vi "NI5112.ProcCases.vi"(0 "i ref in":refnum<vi>, 1 "selector":string, 2 "Data":T1, 3 "call cluster":T2={"Object"="", "Selector"="", "CallType"=enum."synchronous", "Async Object"="", "Async Selector"="", "Data Descriptor"="", "Data"=[], "Error #"=0, "Expire"=0}, 5 "error in (no error)":errorcluster) -> (14 "i ref out":refnum<vi>, 17 "answer cluster":T2={"Object"="", "Selector"="", "CallType"=enum."synchronous", "Async Object"="", "Async Selector"="", "Data Descriptor"="", "Data"=[], "Error #"=0, "Expire"=0}, 19 "error out":errorcluster)   [LabVIEW 2014, in "NI5112.lvlib"]
doc: "This method is called by a process from within the default case in the event loop. The methods of a class that are linked to events will be called from THIS method. Add your code here."
uses:
  NI5112.lvlib
  CS_Core/CSSystem/CoreDefs/CoreDefs.call_type.ctl
  CS_Core/BaseProcess/BaseProcess.descriptor string definition.ctl
  CS_Core/CSSystem/CoreDefs/CoreDefs.rawDataType.ctl
  CS_Core/CSSystem/CoreLib/CoreLib.string 2 byte array.vi
  CS_Core/CSSystem/CoreLib/CoreLib.int 2 byte array.vi
  CS_Core/CSSystem/CoreLib/CoreLib.byte array 2 string.vi
  CS_Core/CSSystem/CoreLib/CoreLib.byte array 2 double.vi
  CS_Core/CSSystem/CoreLib/CoreLib.byte array 2 int.vi
  CS_Core/CSSystem/CoreLib/CoreLib.double 2 byte array.vi
  CS_Core/CSSystem/CoreLib/CoreLib.double array 2 byte array.vi
  CS_Core/BaseProcess/BaseProcess.lvlib
  CS_Core/CSSystem/CoreLib/CoreLib.lvlib
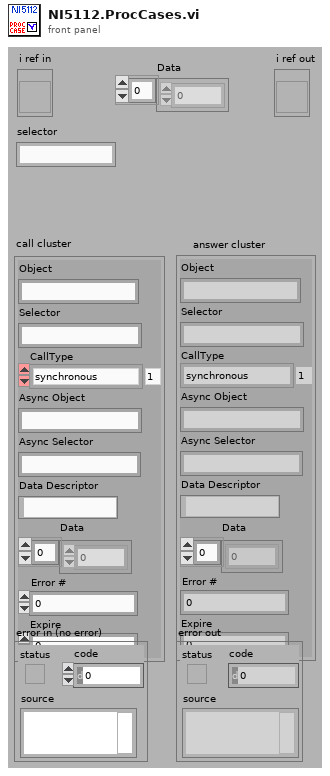
[diagram p1: front panel]
types:
  T1 = typedef "CoreDefs.rawDataType.ctl" = i8[]
  T2 = typedef "CoreDefs.call_type.ctl" = cluster{"Object":string, "Selector":string, "CallType":enum16{"simple", "synchronous", "asynchronous"}, "Async Object":string, "Async Selector":string, "Data Descriptor":T3, "Data":T1, "Error #":i32, "Expire":u32}
  T3 = typedef "BaseProcess.lvlib/BaseProcess.descriptor string definition.ctl" = string
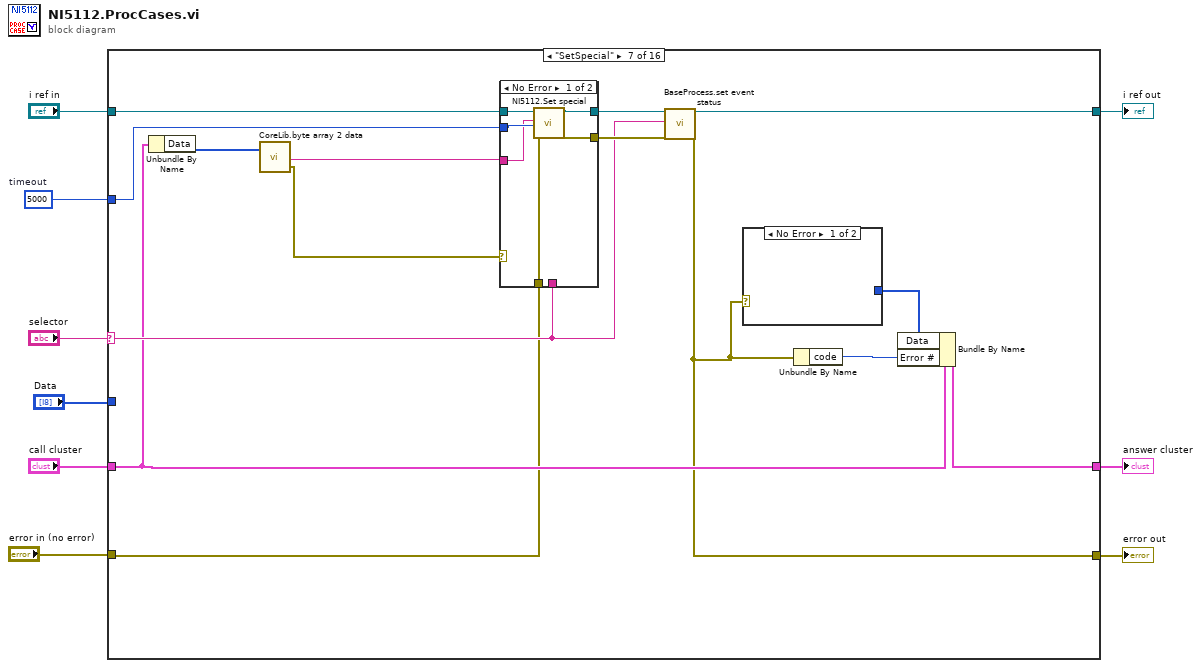
[diagram p0: block diagram]
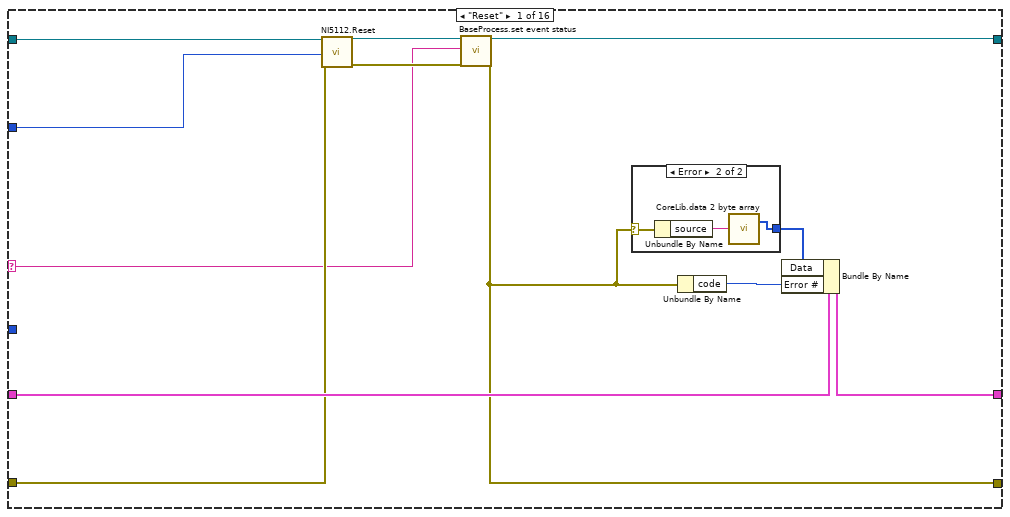
[diagram p2: hidden frame]
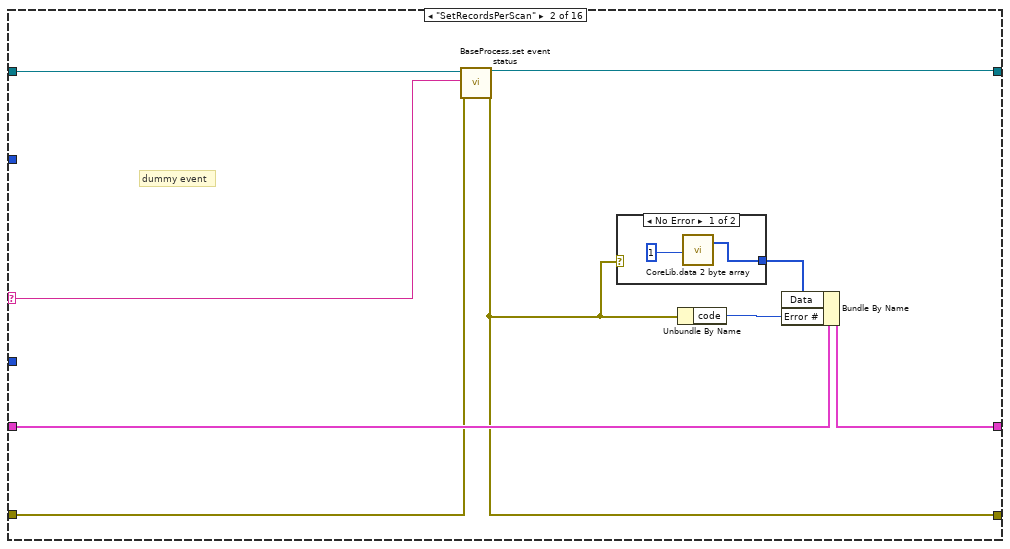
[diagram p4: hidden frame]
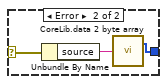
[diagram p5: hidden frame]
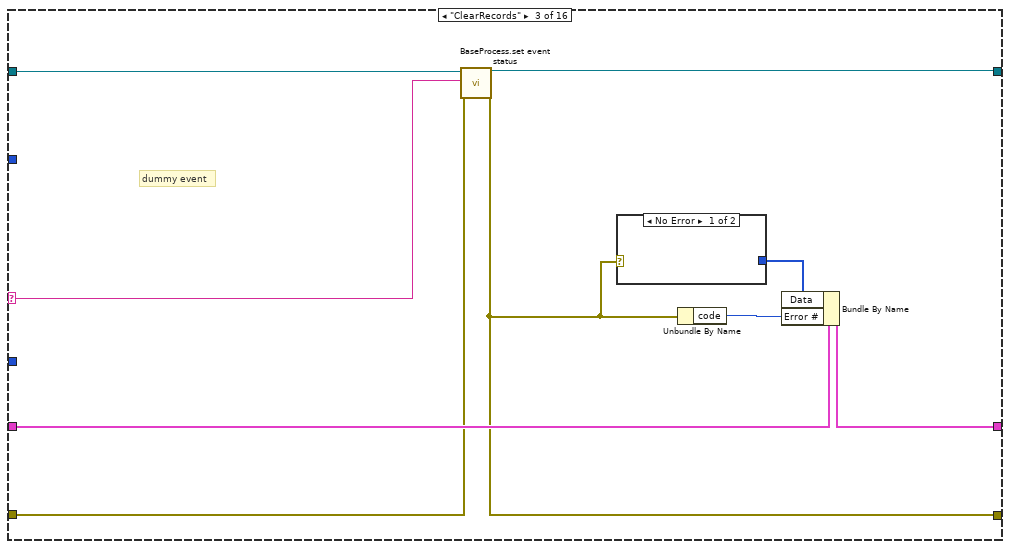
[diagram p6: hidden frame]
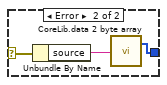
[diagram p7: hidden frame]
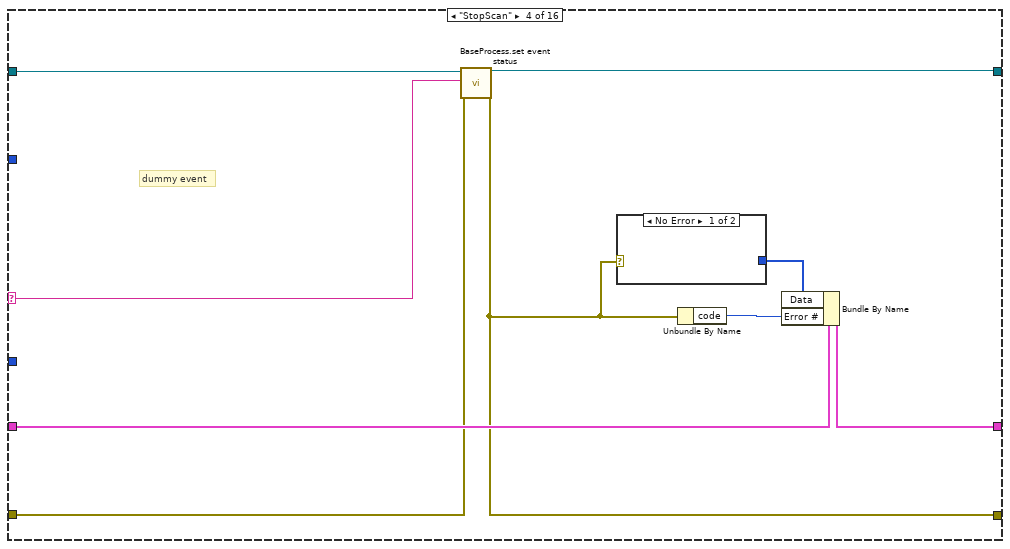
[diagram p8: hidden frame]
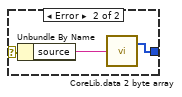
[diagram p9: hidden frame]
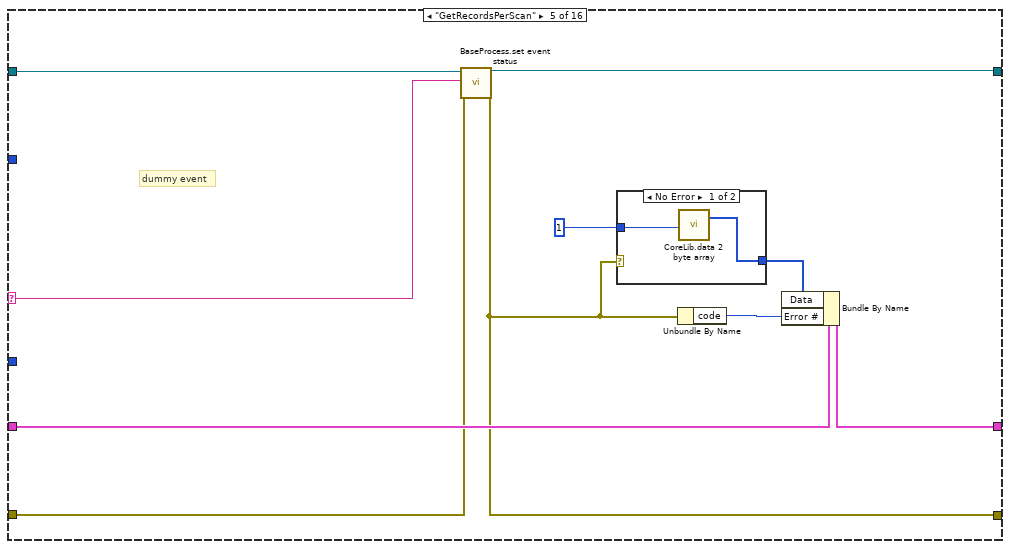
[diagram p10: hidden frame]
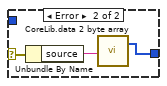
[diagram p11: hidden frame]
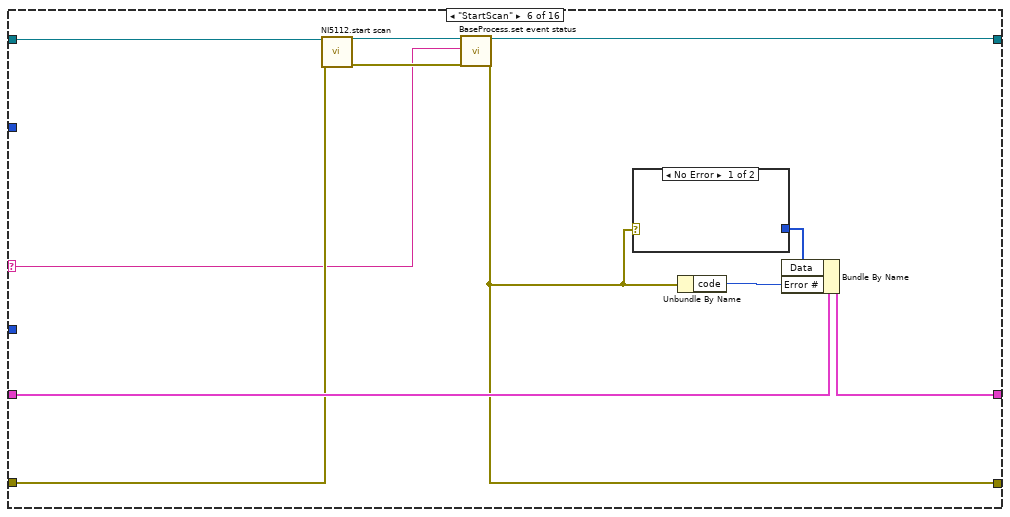
[diagram p12: hidden frame]
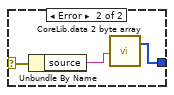
[diagram p13: hidden frame]
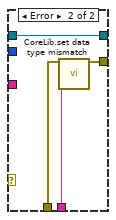
[diagram p14: hidden frame]
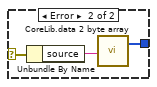
[diagram p15: hidden frame]
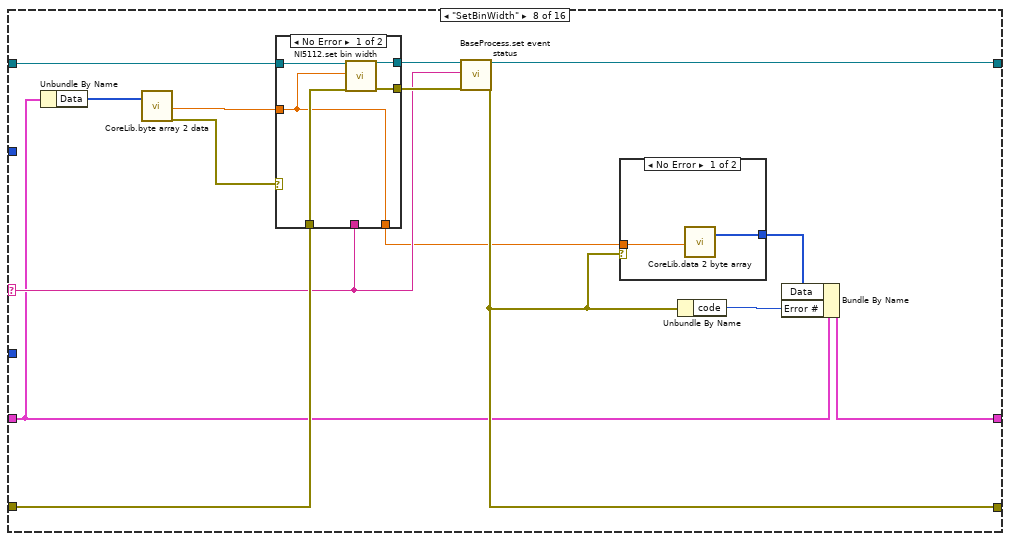
[diagram p16: hidden frame]
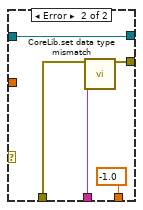
[diagram p17: hidden frame]
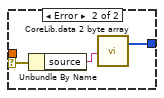
[diagram p18: hidden frame]
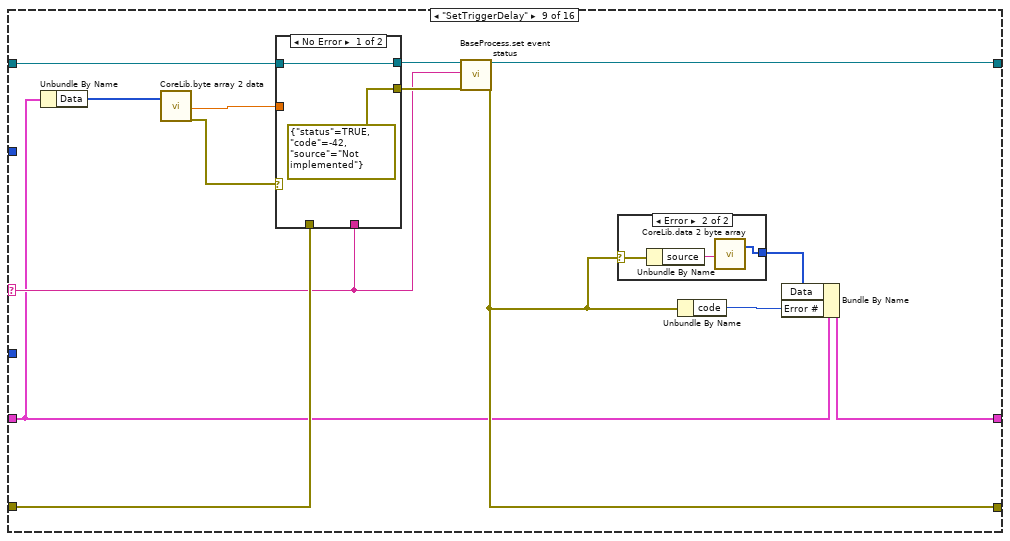
[diagram p19: hidden frame]
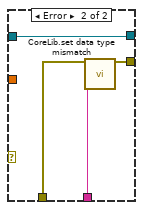
[diagram p20: hidden frame]
diagram:
  w2 = 5000  # timeout
  n1 = case shown="\"SetSpecial\"" "selector" {
    selector: "selector" -> [w11 w26 w40 w52 w65 w78 w100 w125 w154 w178 w205 w223 w243 w265 w282 w298]
    tunnel: "Data" -> [_ _ _ _ _ _ _ _ _ _ _ _ _ _ _ w297]
    tunnel: "i ref in" -> [w17 w25 w39 w51 w64 w84 w102 w131 w160 w184 w211 w229 w249 w271 w288 w304]
    tunnel: [w14 w29 w43 w55 w68 w81 w101 w128 w157 w181 w208 w226 w246 w268 w285 w303] -> w8
    tunnel: "call cluster" -> [w21 w33 w47 w59 w72 w88 w99 w124 w153 w177 w204 w222 w242 w264 w281 w299]
    tunnel: [w20 w32 w46 w58 w71 w87 w96 w134 w163 w187 w214 w232 w251 w274 w291 w300] -> w4
    tunnel: "error in (no error)" -> [w16 w28 w42 w54 w67 w83 w98 w130 w159 w183 w210 w228 w248 w270 w287 w302]
    tunnel: [w12 w27 w41 w53 w66 w79 w97 w126 w155 w179 w206 w224 w244 w266 w283 w301] -> w3
    tunnel: w2 -> [w10 _ _ _ _ _ w95 _ _ _ _ _ _ _ _ _]
    frame "Reset" {
      n2 = call "NI5112.Reset.vi"("i ref in"=w17, "ms timeout (100)"=w10, "error in (no error)"=w16) -> ("i ref out"=w15:refnum<vi>, "error out"=w13:errorcluster)  [unwired: 14 in, 1 out]
      n3 = call "BaseProcess.set event status.vi"("i ref in"=w15, "EventStatus"=w11, "error in (no error)"=w13) -> ("i ref out"=w14:refnum<vi>, "error out"=w12:errorcluster)  [unwired: 14 in, 1 out]
      n4 = case shown="Error" w12 {
        selector: w12 -> [_ w24]
        tunnel: [_ w22] -> w18
        frame No Error {
        }
        frame Error {
          n5 = Unbundle By Name(w24) -> ("source"=w23:string)
          n6 = call-poly "CoreLib.data 2 byte array.vi"("string"=w23) -> ("byteArray out"=w22:T1)  [unwired: 18 in]
        }
      }
      n7 = Unbundle By Name(w12) -> ("code"=w19:i32)
      n8 = Bundle By Name(cluster=w21, "Data"=w18, "Error #"=w19) -> (w20:T2)
    }
    frame "SetRecordsPerScan" {
      # "dummy event"
      n9 = call "BaseProcess.set event status.vi"("i ref in"=w25, "EventStatus"=w26, "error in (no error)"=w28) -> ("i ref out"=w29:refnum<vi>, "error out"=w27:errorcluster)  [unwired: 14 in, 1 out]
      n10 = case shown="No Error" w27 {
        selector: w27 -> [_ w38]
        tunnel: [w34 w36] -> w30
        frame No Error {
          n11 = call-poly "CoreLib.data 2 byte array.vi"("i32"=1) -> ("byteArray out"=w34:T1)  [unwired: 18 in]
        }
        frame Error {
          n12 = Unbundle By Name(w38) -> ("source"=w37:string)
          n13 = call-poly "CoreLib.data 2 byte array.vi"("string"=w37) -> ("byteArray out"=w36:T1)  [unwired: 18 in]
        }
      }
      n14 = Unbundle By Name(w27) -> ("code"=w31:i32)
      n15 = Bundle By Name(cluster=w33, "Data"=w30, "Error #"=w31) -> (w32:T2)
    }
    frame "ClearRecords" {
      # "dummy event"
      n16 = call "BaseProcess.set event status.vi"("i ref in"=w39, "EventStatus"=w40, "error in (no error)"=w42) -> ("i ref out"=w43:refnum<vi>, "error out"=w41:errorcluster)  [unwired: 14 in, 1 out]
      n17 = case shown="No Error" w41 {
        selector: w41 -> [_ w50]
        tunnel: [_ w48] -> w44
        frame No Error {
        }
        frame Error {
          n18 = Unbundle By Name(w50) -> ("source"=w49:string)
          n19 = call-poly "CoreLib.data 2 byte array.vi"("string"=w49) -> ("byteArray out"=w48:T1)  [unwired: 18 in]
        }
      }
      n20 = Unbundle By Name(w41) -> ("code"=w45:i32)
      n21 = Bundle By Name(cluster=w47, "Data"=w44, "Error #"=w45) -> (w46:T2)
    }
    frame "StopScan" {
      # "dummy event"
      n22 = call "BaseProcess.set event status.vi"("i ref in"=w51, "EventStatus"=w52, "error in (no error)"=w54) -> ("i ref out"=w55:refnum<vi>, "error out"=w53:errorcluster)  [unwired: 14 in, 1 out]
      n23 = case shown="No Error" w53 {
        selector: w53 -> [_ w62]
        tunnel: [_ w60] -> w56
        frame No Error {
        }
        frame Error {
          n24 = Unbundle By Name(w62) -> ("source"=w61:string)
          n25 = call-poly "CoreLib.data 2 byte array.vi"("string"=w61) -> ("byteArray out"=w60:T1)  [unwired: 18 in]
        }
      }
      n26 = Unbundle By Name(w53) -> ("code"=w57:i32)
      n27 = Bundle By Name(cluster=w59, "Data"=w56, "Error #"=w57) -> (w58:T2)
    }
    frame "GetRecordsPerScan" {
      # "dummy event"
      n28 = call "BaseProcess.set event status.vi"("i ref in"=w64, "EventStatus"=w65, "error in (no error)"=w67) -> ("i ref out"=w68:refnum<vi>, "error out"=w66:errorcluster)  [unwired: 14 in, 1 out]
      n29 = case shown="No Error" w66 {
        selector: w66 -> [_ w77]
        tunnel: [w73 w75] -> w69
        tunnel: 1 -> [w74 _]
        frame No Error {
          n30 = call-poly "CoreLib.data 2 byte array.vi"("i32"=w74) -> ("byteArray out"=w73:T1)  [unwired: 18 in]
        }
        frame Error {
          n31 = Unbundle By Name(w77) -> ("source"=w76:string)
          n32 = call-poly "CoreLib.data 2 byte array.vi"("string"=w76) -> ("byteArray out"=w75:T1)  [unwired: 18 in]
        }
      }
      n33 = Unbundle By Name(w66) -> ("code"=w70:i32)
      n34 = Bundle By Name(cluster=w72, "Data"=w69, "Error #"=w70) -> (w71:T2)
    }
    frame "StartScan" {
      n35 = call "NI5112.start scan.vi"("i ref in"=w84, "error in (no error)"=w83) -> ("i ref out"=w82:refnum<vi>, "error out"=w80:errorcluster)  [unwired: 15 in, 1 out]
      n36 = call "BaseProcess.set event status.vi"("i ref in"=w82, "EventStatus"=w78, "error in (no error)"=w80) -> ("i ref out"=w81:refnum<vi>, "error out"=w79:errorcluster)  [unwired: 14 in, 1 out]
      n37 = case shown="No Error" w79 {
        selector: w79 -> [_ w91]
        tunnel: [_ w89] -> w85
        frame No Error {
        }
        frame Error {
          n38 = Unbundle By Name(w91) -> ("source"=w90:string)
          n39 = call-poly "CoreLib.data 2 byte array.vi"("string"=w90) -> ("byteArray out"=w89:T1)  [unwired: 18 in]
        }
      }
      n40 = Unbundle By Name(w79) -> ("code"=w86:i32)
      n41 = Bundle By Name(cluster=w88, "Data"=w85, "Error #"=w86) -> (w87:T2)
    }
    frame "SetSpecial" {
      n42 = Unbundle By Name(w99) -> ("Data"=w94:T1)
      n43 = call-poly "CoreLib.byte array 2 data.vi"("byteArray"=w94) -> ("string"=w93:string, "error out"=w92:errorcluster)  [unwired: 16 in, 1 out]
      n44 = case shown="No Error" w92 {
        tunnel: w98 -> [w110 w115]
        tunnel: [w111 w113] -> w104
        tunnel: [w112 w116] -> w103
        tunnel: w100 -> [_ w114]
        tunnel: w93 -> [w107 _]
        tunnel: w95 -> [w109 _]
        tunnel: w102 -> [w108 w113]
        frame No Error {
          n45 = call "NI5112.Set special.vi"("i ref in"=w108, "Special"=w107, "ms timeout (100)"=w109, "error in (no error)"=w110) -> ("i ref out"=w111:refnum<vi>, "error out"=w112:errorcluster)  [unwired: 13 in, 1 out]
        }
        frame Error {
          n46 = call "CoreLib.set data type mismatch.vi"("error in (no error)"=w115, "error source"=w114) -> ("error out"=w116:errorcluster)  [unwired: 17 in]
        }
      }
      n47 = call "BaseProcess.set event status.vi"("i ref in"=w104, "EventStatus"=w100, "error in (no error)"=w103) -> ("i ref out"=w101:refnum<vi>, "error out"=w97:errorcluster)  [unwired: 14 in, 1 out]
      n48 = case shown="No Error" w97 {
        selector: w97 -> [_ w119]
        tunnel: [_ w117] -> w105
        frame No Error {
        }
        frame Error {
          n49 = Unbundle By Name(w119) -> ("source"=w118:string)
          n50 = call-poly "CoreLib.data 2 byte array.vi"("string"=w118) -> ("byteArray out"=w117:T1)  [unwired: 18 in]
        }
      }
      n51 = Unbundle By Name(w97) -> ("code"=w106:i32)
      n52 = Bundle By Name(cluster=w99, "Data"=w105, "Error #"=w106) -> (w96:T2)
    }
    frame "SetBinWidth" {
      n53 = Unbundle By Name(w124) -> ("Data"=w120:T1)
      n54 = call-poly "CoreLib.byte array 2 data.vi"("byteArray"=w120) -> ("d64"=w122:dbl, "error out"=w121:errorcluster)  [unwired: 16 in, 1 out]
      n55 = case shown="No Error" w121 {
        tunnel: w131 -> [w139 w141]
        tunnel: w130 -> [w138 w143]
        tunnel: [w137 w141] -> w129
        tunnel: [w136 w144] -> w127
        tunnel: w125 -> [_ w142]
        tunnel: w122 -> [w135 _]
        tunnel: [w135 -1.0 ("act bin width")] -> w123
        frame No Error {
          n56 = call "NI5112.set bin width.vi"("i ref in"=w139, "bin width [us]"=w135, "error in (no error)"=w138) -> ("i ref out"=w137:refnum<vi>, "error out"=w136:errorcluster)  [unwired: 14 in, 1 out]
        }
        frame Error {
          n57 = call "CoreLib.set data type mismatch.vi"("error in (no error)"=w143, "error source"=w142) -> ("error out"=w144:errorcluster)  [unwired: 17 in]
        }
      }
      n58 = call "BaseProcess.set event status.vi"("i ref in"=w129, "EventStatus"=w125, "error in (no error)"=w127) -> ("i ref out"=w128:refnum<vi>, "error out"=w126:errorcluster)  [unwired: 14 in, 1 out]
      n59 = case shown="No Error" w126 {
        selector: w126 -> [_ w149]
        tunnel: [w145 w148] -> w132
        tunnel: w123 -> [w146 _]
        frame No Error {
          n60 = call-poly "CoreLib.data 2 byte array.vi"("i32"=w146) -> ("byteArray out"=w145:T1)  [unwired: 18 in]
        }
        frame Error {
          n61 = Unbundle By Name(w149) -> ("source"=w147:string)
          n62 = call-poly "CoreLib.data 2 byte array.vi"("string"=w147) -> ("byteArray out"=w148:T1)  [unwired: 18 in]
        }
      }
      n63 = Unbundle By Name(w126) -> ("code"=w133:i32)
      n64 = Bundle By Name(cluster=w124, "Data"=w132, "Error #"=w133) -> (w134:T2)
    }
    frame "SetTriggerDelay" {
      n65 = Unbundle By Name(w153) -> ("Data"=w151:T1)
      n66 = call-poly "CoreLib.byte array 2 data.vi"("byteArray"=w151) -> ("d64"=w152:dbl, "error out"=w150:errorcluster)  [unwired: 16 in, 1 out]
      n67 = case shown="No Error" w150 {
        tunnel: w160 -> [w164 w166]
        tunnel: w159 -> [_ w168]
        tunnel: [w164 w166] -> w158
        tunnel: [errorcluster {"status"=TRUE, "code"=-42, "source"="Not implemented"} ("error out") w169] -> w156
        tunnel: w154 -> [_ w167]
        tunnel: w152 -> [_ _]
        frame No Error {
        }
        frame Error {
          n68 = call "CoreLib.set data type mismatch.vi"("error in (no error)"=w168, "error source"=w167) -> ("error out"=w169:errorcluster)  [unwired: 17 in]
        }
      }
      n69 = call "BaseProcess.set event status.vi"("i ref in"=w158, "EventStatus"=w154, "error in (no error)"=w156) -> ("i ref out"=w157:refnum<vi>, "error out"=w155:errorcluster)  [unwired: 14 in, 1 out]
      n70 = case shown="Error" w155 {
        selector: w155 -> [_ w172]
        tunnel: [_ w170] -> w161
        frame No Error {
        }
        frame Error {
          n71 = Unbundle By Name(w172) -> ("source"=w171:string)
          n72 = call-poly "CoreLib.data 2 byte array.vi"("string"=w171) -> ("byteArray out"=w170:T1)  [unwired: 18 in]
        }
      }
      n73 = Unbundle By Name(w155) -> ("code"=w162:i32)
      n74 = Bundle By Name(cluster=w153, "Data"=w161, "Error #"=w162) -> (w163:T2)
    }
    frame "SetBinsPerRecord" {
      n75 = Unbundle By Name(w177) -> ("Data"=w175:T1)
      n76 = call-poly "CoreLib.byte array 2 data.vi"("byteArray"=w175) -> ("i32"=w174:i32, "error out"=w173:errorcluster)  [unwired: 16 in, 1 out]
      n77 = case shown="No Error" w173 {
        tunnel: w184 -> [w192 w194]
        tunnel: w183 -> [w191 w196]
        tunnel: [w190 w194] -> w182
        tunnel: [w189 w197] -> w180
        tunnel: w178 -> [_ w195]
        tunnel: w174 -> [w188 _]
        tunnel: [w188 -1 ("act bins per recored")] -> w176
        frame No Error {
          n78 = call "NI5112.SetBinsPerRecord.vi"("i ref in"=w192, "bins per record"=w188, "error in (no error)"=w191) -> ("i ref out"=w190:refnum<vi>, "error out"=w189:errorcluster)  [unwired: 14 in, 1 out]
        }
        frame Error {
          n79 = call "CoreLib.set data type mismatch.vi"("error in (no error)"=w196, "error source"=w195) -> ("error out"=w197:errorcluster)  [unwired: 17 in]
        }
      }
      n80 = call "BaseProcess.set event status.vi"("i ref in"=w182, "EventStatus"=w178, "error in (no error)"=w180) -> ("i ref out"=w181:refnum<vi>, "error out"=w179:errorcluster)  [unwired: 14 in, 1 out]
      n81 = case shown="No Error" w179 {
        selector: w179 -> [_ w202]
        tunnel: [w198 w200] -> w185
        tunnel: w176 -> [w199 _]
        frame No Error {
          n82 = call-poly "CoreLib.data 2 byte array.vi"("i32"=w199) -> ("byteArray out"=w198:T1)  [unwired: 18 in]
        }
        frame Error {
          n83 = Unbundle By Name(w202) -> ("source"=w201:string)
          n84 = call-poly "CoreLib.data 2 byte array.vi"("string"=w201) -> ("byteArray out"=w200:T1)  [unwired: 18 in]
        }
      }
      n85 = Unbundle By Name(w179) -> ("code"=w186:i32)
      n86 = Bundle By Name(cluster=w177, "Data"=w185, "Error #"=w186) -> (w187:T2)
    }
    frame "GetScanStatus" {
      n87 = call "NI5112.get scan status.vi"("i ref in"=w211, "error in (no error)"=w210) -> ("i ref out"=w209:refnum<vi>, "x != y?"=w203:bool, "error out"=w207:errorcluster)  [unwired: 14 in, 1 out]
      n88 = call "BaseProcess.set event status.vi"("i ref in"=w209, "EventStatus"=w205, "error in (no error)"=w207) -> ("i ref out"=w208:refnum<vi>, "error out"=w206:errorcluster)  [unwired: 14 in, 1 out]
      n89 = case shown="No Error" w206 {
        selector: w206 -> [_ w220]
        tunnel: [w215 w218] -> w212
        tunnel: w203 -> [w217 _]
        frame No Error {
          n90 = Flatten To String(anything=w217) -> (data string=w216:string)  [unwired: 3 in, 2 out]
          n91 = call-poly "CoreLib.data 2 byte array.vi"("string"=w216) -> ("byteArray out"=w215:T1)  [unwired: 18 in]
        }
        frame Error {
          n92 = Unbundle By Name(w220) -> ("source"=w219:string)
          n93 = call-poly "CoreLib.data 2 byte array.vi"("string"=w219) -> ("byteArray out"=w218:T1)  [unwired: 18 in]
        }
      }
      n94 = Unbundle By Name(w206) -> ("code"=w213:i32)
      n95 = Bundle By Name(cluster=w204, "Data"=w212, "Error #"=w213) -> (w214:T2)
    }
    frame "GetBinData" {
      n96 = call "NI5112.get bin data.vi"("i ref in"=w229, "error in (no error)"=w228) -> ("i ref out"=w227:refnum<vi>, "Output Waveform"=w221:waveform(dbl), "error out"=w225:errorcluster)  [unwired: 14 in, 1 out]
      n97 = call "BaseProcess.set event status.vi"("i ref in"=w227, "EventStatus"=w223, "error in (no error)"=w225) -> ("i ref out"=w226:refnum<vi>, "error out"=w224:errorcluster)  [unwired: 14 in, 1 out]
      n98 = case shown="No Error" w224 {
        selector: w224 -> [_ w238]
        tunnel: [w234 w237] -> w230
        tunnel: w221 -> [w235 _]
        frame No Error {
          n99 = Flatten To String(anything=w235) -> (data string=w233:string)  [unwired: 3 in, 2 out]
          n100 = call-poly "CoreLib.data 2 byte array.vi"("string"=w233) -> ("byteArray out"=w234:T1)  [unwired: 18 in]
        }
        frame Error {
          n101 = Unbundle By Name(w238) -> ("source"=w236:string)
          n102 = call-poly "CoreLib.data 2 byte array.vi"("string"=w236) -> ("byteArray out"=w237:T1)  [unwired: 18 in]
        }
      }
      n103 = Unbundle By Name(w224) -> ("code"=w231:i32)
      n104 = Bundle By Name(cluster=w222, "Data"=w230, "Error #"=w231) -> (w232:T2)
    }
    frame "ReadData" {
      n105 = call "NI5112.get bin data.vi"("i ref in"=w249, "error in (no error)"=w248) -> ("i ref out"=w247:refnum<vi>, "Output Waveform"=w239:waveform(dbl), "error out"=w245:errorcluster)  [unwired: 14 in, 1 out]
      n106 = call "BaseProcess.set event status.vi"("i ref in"=w247, "EventStatus"=w243, "error in (no error)"=w245) -> ("i ref out"=w246:refnum<vi>, "error out"=w244:errorcluster)  [unwired: 14 in, 1 out]
      n107 = case shown="No Error" w244 {
        selector: w244 -> [_ w262]
        tunnel: [w257 w260] -> w241
        tunnel: w239 -> [w259 _]
        frame No Error {
          n108 = Unbundle By Name(w259) -> ("t0"=w258:timestamp, "dt"=w253:dbl, "Y"=w252:dbl[])
          n109 = To Double Precision Float(number=w258) -> (double precision float=w254:dbl)
          n110 = call-poly "CoreLib.data 2 byte array.vi"("f64"=w254) -> ("byteArray out"=w255:T1)  [unwired: 18 in]
          n111 = call-poly "CoreLib.data 2 byte array.vi"("byteArray"=w255, "f64"=w253) -> ("byteArray out"=w256:T1)  [unwired: 17 in]
          n112 = call-poly "CoreLib.data 2 byte array.vi"("byteArray"=w256, "[d64]"=w252) -> ("byteArray out"=w257:T1)  [unwired: 17 in]
        }
        frame Error {
          n113 = Unbundle By Name(w262) -> ("source"=w261:string)
          n114 = call-poly "CoreLib.data 2 byte array.vi"("string"=w261) -> ("byteArray out"=w260:T1)  [unwired: 18 in]
        }
      }
      n115 = Unbundle By Name(w244) -> ("code"=w250:i32)
      n116 = Bundle By Name(cluster=w242, "Data"=w241, "Error #"=w250, "Data Descriptor"=T3 "D:1;D:1;D:N") -> (w251:T2)
    }
    frame "GetBinWidth" {
      n117 = call "NI5112.get bin width.vi"("i ref in"=w271, "error in (no error)"=w270) -> ("i ref out"=w269:refnum<vi>, "bin width (us)"=w263:dbl, "error out"=w267:errorcluster)  [unwired: 14 in, 1 out]
      n118 = call "BaseProcess.set event status.vi"("i ref in"=w269, "EventStatus"=w265, "error in (no error)"=w267) -> ("i ref out"=w268:refnum<vi>, "error out"=w266:errorcluster)  [unwired: 14 in, 1 out]
      n119 = case shown="No Error" w266 {
        selector: w266 -> [_ w279]
        tunnel: [w275 w278] -> w272
        tunnel: w263 -> [w276 _]
        frame No Error {
          n120 = call-poly "CoreLib.data 2 byte array.vi"("f64"=w276) -> ("byteArray out"=w275:T1)  [unwired: 18 in]
        }
        frame Error {
          n121 = Unbundle By Name(w279) -> ("source"=w277:string)
          n122 = call-poly "CoreLib.data 2 byte array.vi"("string"=w277) -> ("byteArray out"=w278:T1)  [unwired: 18 in]
        }
      }
      n123 = Unbundle By Name(w266) -> ("code"=w273:i32)
      n124 = Bundle By Name(cluster=w264, "Data"=w272, "Error #"=w273) -> (w274:T2)
    }
    frame "GetBinsPerRecord" {
      n125 = call "NI5112.get bins per record.vi"("i ref in"=w288, "error in (no error)"=w287) -> ("i ref out"=w286:refnum<vi>, "binsperrecord"=w280:i32, "error out"=w284:errorcluster)  [unwired: 14 in, 1 out]
      n126 = call "BaseProcess.set event status.vi"("i ref in"=w286, "EventStatus"=w282, "error in (no error)"=w284) -> ("i ref out"=w285:refnum<vi>, "error out"=w283:errorcluster)  [unwired: 14 in, 1 out]
      n127 = case shown="No Error" w283 {
        selector: w283 -> [_ w296]
        tunnel: [w292 w294] -> w289
        tunnel: w280 -> [w293 _]
        frame No Error {
          n128 = call-poly "CoreLib.data 2 byte array.vi"("i32"=w293) -> ("byteArray out"=w292:T1)  [unwired: 18 in]
        }
        frame Error {
          n129 = Unbundle By Name(w296) -> ("source"=w295:string)
          n130 = call-poly "CoreLib.data 2 byte array.vi"("string"=w295) -> ("byteArray out"=w294:T1)  [unwired: 18 in]
        }
      }
      n131 = Unbundle By Name(w283) -> ("code"=w290:i32)
      n132 = Bundle By Name(cluster=w281, "Data"=w289, "Error #"=w290) -> (w291:T2)
    }
    frame Default {
      n133 = call "BaseProcess.ProcCases.vi"("i ref in"=w304, "selector"=w298, "Data"=w297, "call cluster"=w299, "error in (no error)"=w302) -> ("i ref out"=w303:refnum<vi>, "answer cluster"=w300:T2, "error out"=w301:errorcluster)  [unwired: 12 in]
    }
  }
  "answer cluster" <- w4
  "i ref out" <- w8
  "error out" <- w3
